vi "Save Data File.vi"(0 "File Type":T1, 1 "Data":dbl[](array[numeric]), 2 "Open File Location":bool, 3 "error in (no error)":errorcluster) -> (10 "error out":errorcluster)   [LabVIEW 2018]
uses:
  <vilib>/Utility/TDMS File Viewer/NI_TDMS File Viewer.lvlib
  controls/File Type.ctl
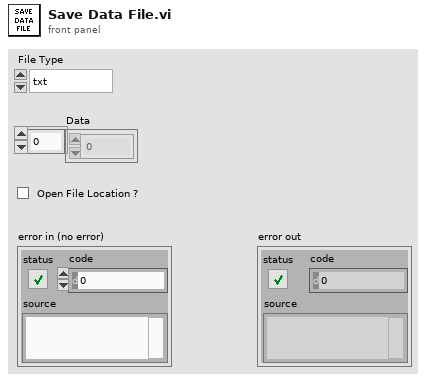
[diagram p1: front panel]
types:
  T1 = typedef "File Type.ctl" = enum16{"txt", "csv", "tdms"}
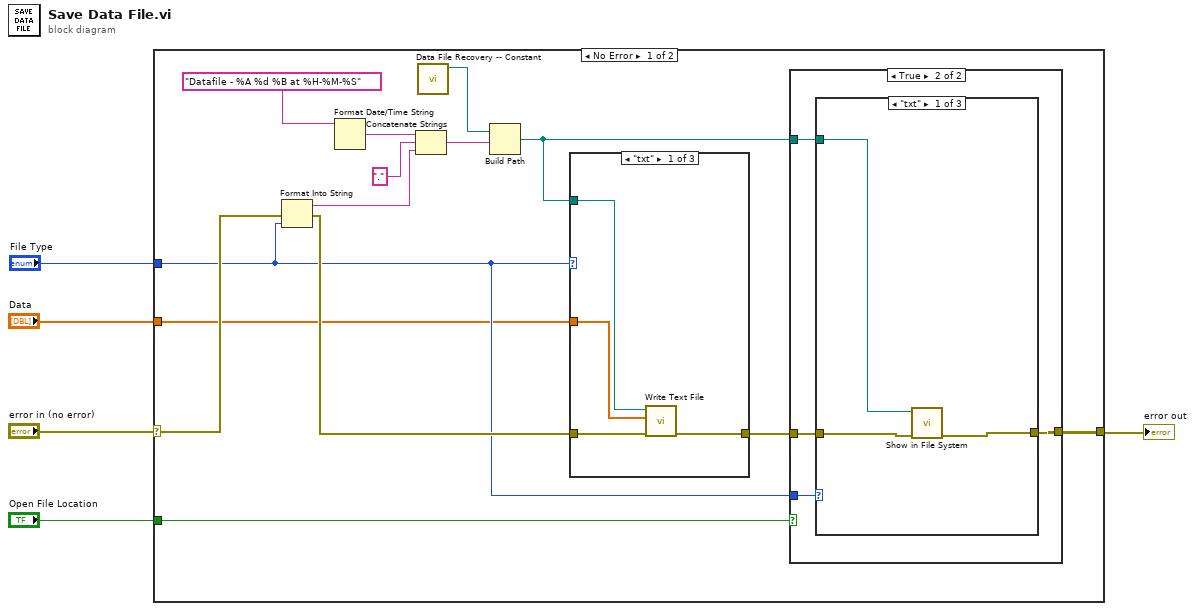
[diagram p0: block diagram]
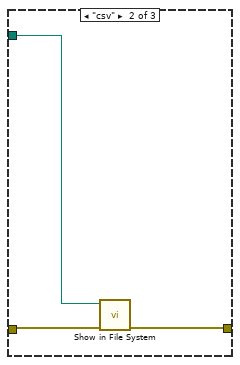
[diagram p3: hidden frame]
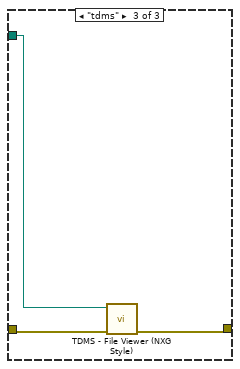
[diagram p4: hidden frame]
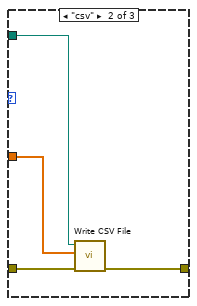
[diagram p5: hidden frame]
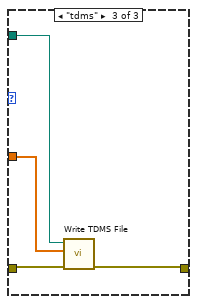
[diagram p6: hidden frame]
diagram:
  n1 = case shown="No Error" "error in (no error)" {
    selector: "error in (no error)" -> [w16 w46]
    tunnel: [w6 w46] -> w4
    tunnel: "Data" -> [w7 _]
    tunnel: "Open File Location" -> [w10 _]
    tunnel: "File Type" -> [w11 _]
    frame No Error {
      n2 = Format Into String(error in=w16, w11) -> (resulting string=w15:string, error out=w12:errorcluster)  [unwired: 2 in]
      n3 = Format Date/Time String(time format string (%c)="Datafile - %A %d %B at %H-%M-%S") -> (date/time string=w18:string)  [unwired: 2 in]
      n4 = Concatenate Strings(w18, "." ("string"), w15) -> (w14:string)
      n5 = call "Data File Recovery -- Constant.vi"() -> ("Data File Directory"=w13:path)  [unwired: 11 in]
      n6 = Build Path(base path=w13, name or relative path=w14) -> (appended path=w9:path)
      n7 = case shown="\"txt\"" w11 {
        tunnel: w12 -> [w36 w40 w44]
        tunnel: w9 -> [w35 w39 w42]
        tunnel: [w37 w41 w45] -> w8
        tunnel: w7 -> [w34 w38 w43]
        frame "txt" {
          n8 = call "Write Text File.vi"("error in (no error)"=w36, "Data"=w34, "Path"=w35) -> ("error out"=w37:errorcluster)  [unwired: 8 in]
        }
        frame "csv" {
          n9 = call "Write CSV File.vi"("error in (no error)"=w40, "Data"=w38, "Path"=w39) -> ("error out"=w41:errorcluster)  [unwired: 8 in]
        }
        frame "tdms" {
          n10 = call "Write TDMS File.vi"("error in (no error)"=w44, "Data"=w43, "Path"=w42) -> ("error out"=w45:errorcluster)  [unwired: 8 in]
        }
      }
      n11 = case shown="True" w10 {
        tunnel: w11 -> [_ w24]
        tunnel: w9 -> [_ w23]
        tunnel: w8 -> [w20 w22]
        tunnel: [w20 w21] -> w6
        frame False {
        }
        frame True {
          n12 = case shown="\"txt\"" w24 {
            tunnel: w23 -> [w25 w28 w31]
            tunnel: w22 -> [w27 w30 w33]
            tunnel: [w26 w29 w32] -> w21
            frame "txt" {
              n13 = call <vilib>:"Show in File System.vi"("error in (no error)"=w27, "file or directory path"=w25) -> ("error out"=w26:errorcluster)  [unwired: 9 in]
            }
            frame "csv" {
              n14 = call <vilib>:"Show in File System.vi"("error in (no error)"=w30, "file or directory path"=w28) -> ("error out"=w29:errorcluster)  [unwired: 9 in]
            }
            frame "tdms" {
              n15 = call <vilib>:"TDMS - File Viewer (NXG Style).vi"("error in"=w33, "file in"=w31) -> ("error out"=w32:errorcluster)  [unwired: 8 in, 1 out]
            }
          }
        }
      }
    }
    frame Error {
    }
  }
  "error out" <- w4
